vi "Non-SD UI Ref.vi"(8 "error in (no error)":errorcluster, 11 "SD Module in":refnum<class "SD Module.lvclass">) -> (0 "error out":errorcluster, 1 "Show SubPanel?":bool, 2 "VI Refnum":refnum<vi>, 3 "SD Module out":refnum<class "SD Module.lvclass">)   [LabVIEW 2011, in "Modules.lvlib" / "SD Module.lvclass"]
uses:
  SD Module.lvclass
  RSI Module/RSI Module_UI.vi
  RSI Module/RSI Module.lvclass
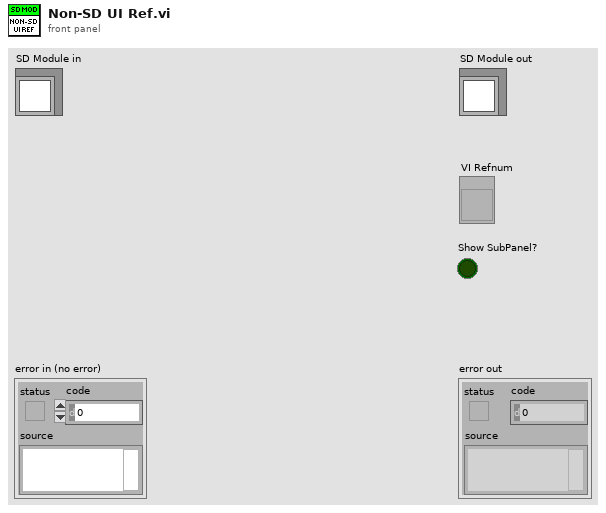
[diagram p1: front panel]
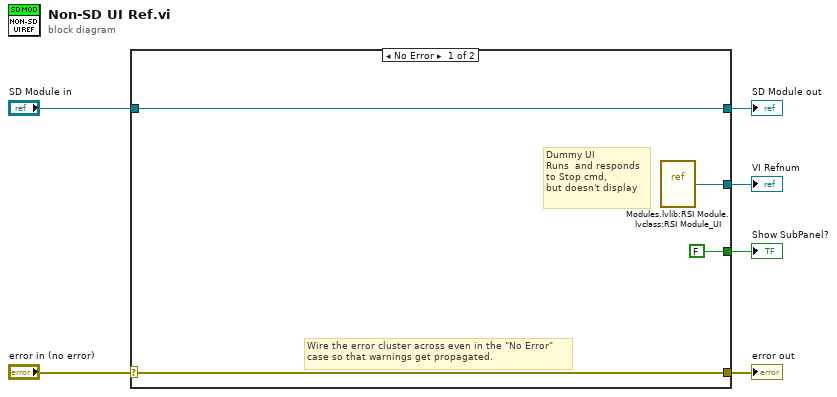
[diagram p0: block diagram]
diagram:
  n1 = case shown="No Error" "error in (no error)" {
    selector: "error in (no error)" -> [w9 w12]
    tunnel: [w9 w12] -> w5
    tunnel: [w10 w11] -> w3
    tunnel: "SD Module in" -> [w10 w11]
    tunnel: [w7 _] -> w2
    tunnel: [FALSE _] -> w1
    frame No Error {
      # "Dummy UI\nRuns  and responds\nto Stop cmd, \nbut doesn't display"
      # "Wire the error cluster across even in the \"No Error\"\ncase so that warnings get propagated."
      n2 = vi-ref "Modules.lvlib:RSI Module.lvclass:RSI Module_UI.vi"() -> (w7:refnum<vi>)
    }
    frame Error {
    }
  }
  "error out" <- w5
  "SD Module out" <- w3
  "VI Refnum" <- w2
  "Show SubPanel?" <- w1
